vi "XYZ mov setup-format and values.vi"() -> (13 "Values.Boolean":bool[](array[boolean]), 14 "Keys setup.DBL":T2=[{"key"="Control FPGA.Clock Freq (MHz)", "Save?"=TRUE, "Default"=240.0}, {"key"="DAQ FPGA.Clock Freq (MHz)", "Save?"=TRUE, "Default"=240.0}], 15 "Values.DBL":dbl[](array[numeric]) format="%#_9f", 16 "Keys setup.String":T3=[{"key"="Control FPGA.MAC address", "Save?"=TRUE, "Default"="AABBCCDDEEFF"}, {"key"="DAQ FPGA.Target", "Save?"=TRUE, "Default"="RIO0"}, {"key"="XY Stage.COM port", "Save?"=TRUE, "Default"="COM7"}, {"key"="DAQmx Chan.Pockels Control", "Save?"=TRUE, "Default"=""}, {"key"="DAQmx Chan.Hard Shutter", "Save?"=TRUE, "Default"=""}, {"key"="DAQmx Chan.PMT 1", "Save?"=TRUE, "Default"=""}, {"key"="DAQmx Chan.PMT 2", "Save?"=TRUE, "Default"=""}, {"key"="DAQmx Chan.Encoder Trigger", "Save?"=TRUE, "Default"=""}, {"key"="DAQmx Chan.Optional Trigger 1", "Save?"=TRUE, "Default"=""}, {"key"="DAQmx Chan.Optional Trigger 2", "Save?"=TRUE, "Default"=""}, {"key"="DAQmx Chan.Optional Trigger 3", "Save?"=TRUE, "Default"=""}], 17 "Values.Strings":string[](array[string]), 18 "Keys setup.Boolean":T1, 19 "error out":errorcluster)   [LabVIEW 2013]
uses:
  Typedefs/Ini file interface (String).ctl
  Typedefs/Ini file interface (DBL).ctl
  Typedefs/Ini file interface (Boolean).ctl
  User Interface/Windows/Position control window/Globals/Pos ctrl window globals.vi
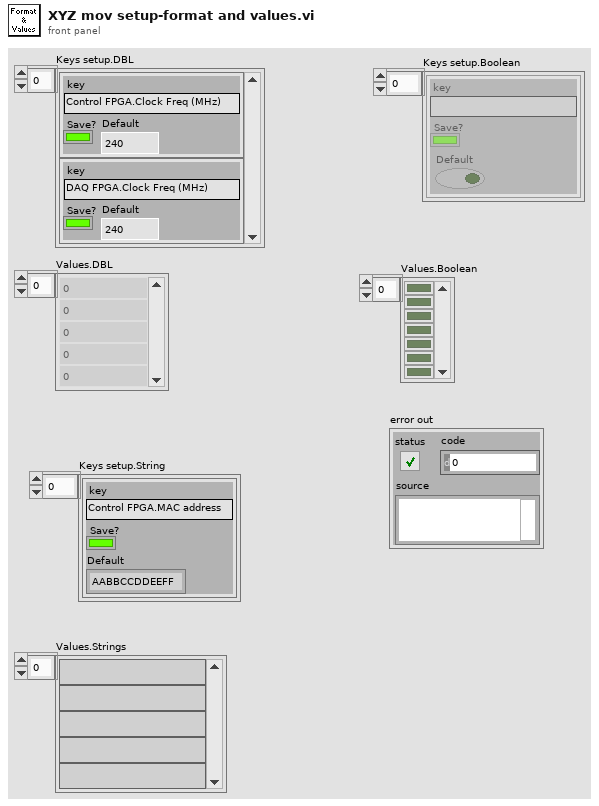
[diagram p1: front panel]
types:
  T1 = typedef "Ini file interface (Boolean).ctl" = cluster{"key":string, "Save?":bool, "Default":bool}[]
  T2 = typedef "Ini file interface (DBL).ctl" = cluster{"key":string, "Save?":bool, "Default":dbl}[]
  T3 = typedef "Ini file interface (String).ctl" = cluster{"key":string, "Save?":bool, "Default":string}[]
  T4 = typedef "Movement mode.ctl" = enum16{"Move the frame", "Move the feature"}
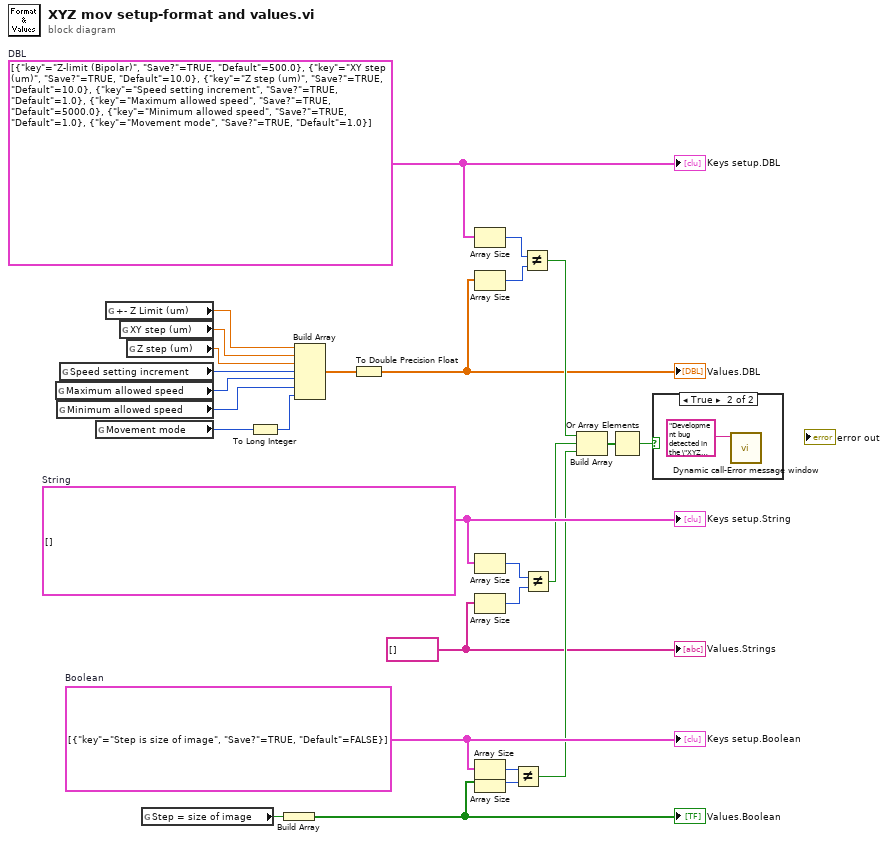
[diagram p0: block diagram]
diagram:
  w1 = string[] [] ("appended array")
  w25 = T1 [{"key"="Step is size of image", "Save?"=TRUE, "Default"=FALSE}]  # Boolean
  w27 = T3 []  # String
  w26 = T2 [{"key"="Z-limit (Bipolar)", "Save?"=TRUE, "Default"=500.0}, {"key"="XY step (um)", "Save?"=TRUE, "Default"=10.0}, {"key"="Z step (um)", "Save?"=TRUE, "Default"=10.0}, {"key"="Speed setting increment", "Save?"=TRUE, "Default"=1.0}, {"key"="Maximum allowed speed", "Save?"=TRUE, "Default"=5000.0}, {"key"="Minimum allowed speed", "Save?"=TRUE, "Default"=1.0}, {"key"="Movement mode", "Save?"=TRUE, "Default"=1.0}]  # DBL
  n1 = global read "Pos ctrl window globals.vi" "Maximum allowed speed"() -> (w11:i32)
  n2 = global read "Pos ctrl window globals.vi" "Minimum allowed speed"() -> (w12:i32)
  n3 = global read "Pos ctrl window globals.vi" "Speed setting increment"() -> (w10:i32)
  n4 = global read "Pos ctrl window globals.vi" "Movement mode"() -> (w9:T4)
  n5 = global read "Pos ctrl window globals.vi" "+- Z Limit (um)"() -> (w5:sgl)
  n6 = global read "Pos ctrl window globals.vi" "XY step (um)"() -> (w6:sgl)
  n7 = global read "Pos ctrl window globals.vi" "Z step (um)"() -> (w7:sgl)
  n8 = global read "Pos ctrl window globals.vi" "Step = size of image"() -> (w2:bool)
  n9 = To Long Integer(number=w9) -> (32bit integer=w8:i32)
  n10 = Build Array(w2) -> (w3:bool[])
  "Values.Boolean" <- w3
  n11 = Build Array(w5, w6, w7, w10, w11, w12, w8) -> (w4:sgl[])
  n12 = To Double Precision Float(number=w4) -> (double precision float=w13:dbl[])
  "Values.DBL" <- w13
  n13 = Array Size(array=w26) -> (size(s)=w22:i32)
  n14 = Array Size(array=w13) -> (size(s)=w21:i32)
  n15 = Array Size(array=w27) -> (size(s)=w24:i32)
  n16 = Array Size(array=w1) -> (size(s)=w23:i32)
  n17 = Array Size(array=w25) -> (size(s)=w20:i32)
  n18 = Array Size(array=w3) -> (size(s)=w19:i32)
  n19 = Not Equal?(x=w20, y=w19) -> (x != y?=w17:bool)
  n20 = Not Equal?(x=w22, y=w21) -> (x != y?=w15:bool)
  n21 = Not Equal?(x=w24, y=w23) -> (x != y?=w14:bool)
  n22 = Build Array(w15, w14, w17) -> (w18:bool[])
  n23 = Or Array Elements(Boolean array=w18) -> (logical OR=w16:bool)
  n24 = case shown="True" w16 {
    frame False {
    }
    frame True {
      n25 = call "Dynamic call-Error message window.vi"("Error Message"="Development bug detected in the \"XYZ mov setup-format and values.vi\".\nPlease correct the set up in this VI.") -> ()  [unwired: 10 in, 1 out]
    }
  }
  "Keys setup.String" <- w27
  "Keys setup.DBL" <- w26
  "Values.Strings" <- w1
  "Keys setup.Boolean" <- w25
